vi "Task Array.vi"() -> ()   [LabVIEW 2024]
uses:
  <vilib>/Analysis/Matrix/Datatypes/RealMatrix.ctl
  <vilib>/Analysis/7linalg.llb/Solve Linear Equations (multiple right hand).vi
  <vilib>/Analysis/NI_AALPro.lvlib
  <vilib>/Analysis/Matrix/NI_Matrix.lvlib
panel:
  out "Solution Matrix 3":T1
  in  "Vectors 3":T1
  in  "Coefficient Array 3":T1
  out "Solution Matrix 2":T1
  in  "Vectors 2":T1
  in  "Coefficient Array 2":T1
  out "Solution Matrix":T1
  in  "Vectors":T1
  in  "Coefficient Array":T1
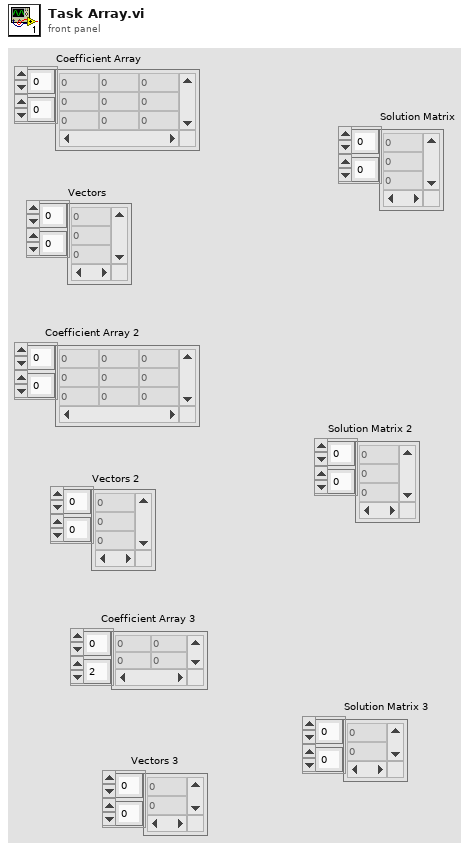
[diagram p1: front panel]
types:
  T1 = typedef "NI_Matrix.lvlib/RealMatrix.ctl" = dbl[][]
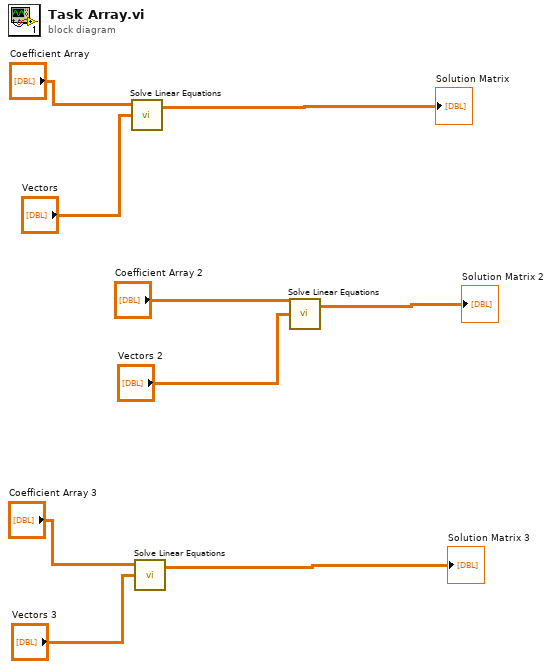
[diagram p0: block diagram]
diagram:
  n1 = call-poly <vilib>:"Solve Linear Equations.vi"("Known Matrix"="Vectors", "Input Matrix"="Coefficient Array") -> ("Solution Matrix"=→"Solution Matrix":T1)  [unwired: 1 in, 1 out]
  n2 = call-poly <vilib>:"Solve Linear Equations.vi"("Known Matrix"="Vectors 3", "Input Matrix"="Coefficient Array 3") -> ("Solution Matrix"=→"Solution Matrix 3":T1)  [unwired: 1 in, 1 out]
  n3 = call-poly <vilib>:"Solve Linear Equations.vi"("Known Matrix"="Vectors 2", "Input Matrix"="Coefficient Array 2") -> ("Solution Matrix"=→"Solution Matrix 2":T1)  [unwired: 1 in, 1 out]
